vi "Fluke 884X Series Read Single Measurement.vi"() -> ()   [LabVIEW 2010]
doc: "This example shows how to configure a measurement and take a single reading."
uses:
  <vilib>/Utility/error.llb/DialogType.ctl
  <instrlib>/Fluke 884X Series/Public/Data/Read (Single Point).vi
  <instrlib>/Fluke 884X Series/Fluke 884X Series.lvlib
panel:
  out "Measurement":dbl
  in  "Manual Range (1.0)":dbl=1.0
  in  "Auto Range (T:Enable)":bool=TRUE
  in  "Manual Resolution (5.5 Digits)":dbl(ring)=5.5 items=["4.5"=4.5, "5.5"=5.5, "6.5"=6.5]
  in  "Function (0: DC Voltage)":u16(ring) items=["DC Voltage", "AC Voltage", "2 - Wire Resistance", "4 - Wire Resistance", "DC Current", "AC Current", "Frequency", "Period", "Continuity", "Diode Checking", "Temperature", "Capacitance"]
  in  "Serial Configuration":T1={"Baud Rate"=9600, "Parity"=0, "Data Bits"=8, "Stop Bits"=10, "Flow Control"=0} {"Flow Control" items=["None", "XON/XOFF", "RTS/CTS", "XON/XOFF & RTS/CTS", "DTR/DSR", "XON/XOFF & DTR/DSR"]; "Stop Bits" items=["1.0"=10, "1.5"=15, "2.0"=20]; "Data Bits" items=["7"=7, "8"=8]; "Parity" items=["None", "Odd", "Even", "Mark", "Space"]; "Baud Rate" items=["300"=300, "600"=600, "1200"=1200, "2400"=2400, "4800"=4800, "9600"=9600, "19200"=19200]}
  in  "VISA resource name":refnum<visa-resource-name>
  # "(c) 2007 National Instruments.  ALL RIGHTS RESERVED."
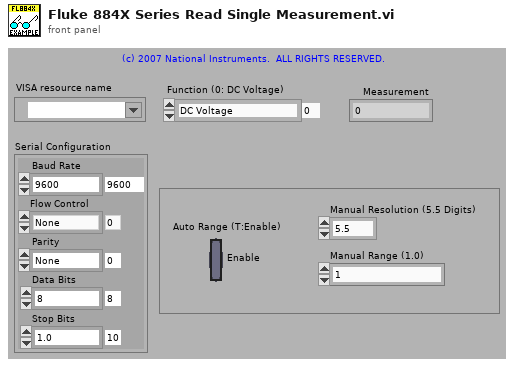
[diagram p1: front panel]
types:
  T1 = cluster{"Baud Rate":u32, "Parity":u16, "Data Bits":u16, "Stop Bits":u16, "Flow Control":u16}
  T2 = typedef "DialogType.ctl" = u16
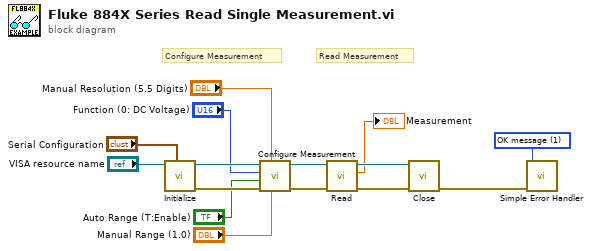
[diagram p0: block diagram]
diagram:
  w10 = T2 1 items=["no dialog", "OK message", "continue or stop message", "OK message + warnings", "continue/stop + warnings"] ("type of dialog (OK msg:1)")
  # "Read Measurement"
  # "Configure Measurement"
  n1 = call <instrlib>:"Initialize.vi"("Serial Configuration"="Serial Configuration", "VISA resource name"="VISA resource name") -> ("error out"=w11:errorcluster, "VISA resource name out"=w12:refnum<visa-resource-name>)  [unwired: 8 in]
  n2 = call <instrlib>:"Configure Measurement.vi"("Manual Range (1.0)"="Manual Range (1.0)", "Manual Resolution (5.5 Digits)"="Manual Resolution (5.5 Digits)", "error in (no error)"=w11, "Auto Range (T:Enable)"="Auto Range (T:Enable)", "Function (0: DC Voltage)"="Function (0: DC Voltage)", "VISA resource name"=w12) -> ("error out"=w1:errorcluster, "VISA resource name out"=w2:refnum<visa-resource-name>)  [unwired: 4 in]
  n3 = call-poly <instrlib>:"Read.vi"("error in (no error)"=w1, "VISA resource name"=w2) -> ("error out"=w14:errorcluster, "Measurement"=→"Measurement":dbl, "VISA resource name out"=w13:refnum<visa-resource-name>)  [unwired: 7 in]
  n4 = call <instrlib>:"Close.vi"("error in (no error)"=w14, "VISA resource name"=w13) -> ("error out"=w15:errorcluster)  [unwired: 9 in]
  n5 = call <vilib>:"Simple Error Handler.vi"("type of dialog (OK msg:1)"=w10, "error in (no error)"=w15) -> ()  [unwired: 3 in, 5 out]
